vi "gcodeTec.vi"() -> ()   [LabVIEW 2025]
panel:
  out "subarray":dbl[][][](array[numeric])
  out "Array":dbl[][][](array[numeric])
  out "string in":string
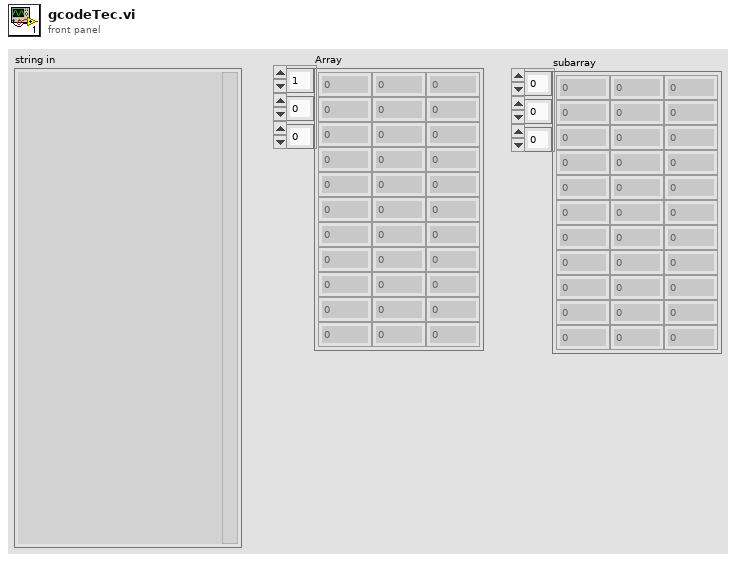
[diagram p1: front panel]
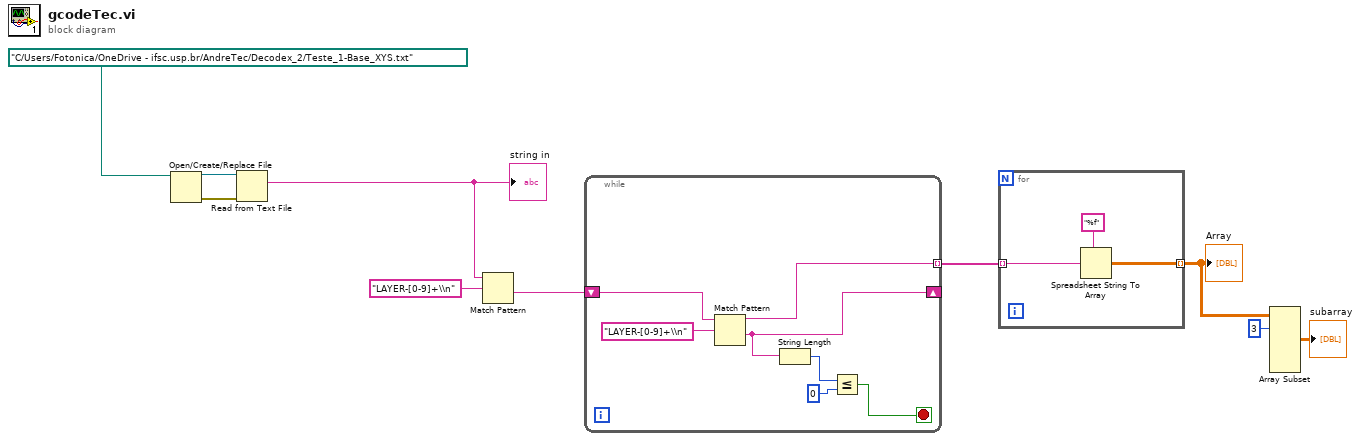
[diagram p0: block diagram]
diagram:
  n1 = Open/Create/Replace File(file path (use dialog)=path "C:/Users/Fotonica/OneDrive - ifsc.usp.br/AndreTec/Decodex_2/Teste_1-Base_XYS.txt") -> (refnum out=w9:refnum<file>, error out=w10:errorcluster)  [unwired: 5 in, 1 out]
  n2 = Read from Text File(file (use dialog)=w9, error in=w10) -> (text=w7:string)  [unwired: 2 in, 3 out]
  "string in" <- w7
  n3 = Match Pattern(string=w7, regular expression="LAYER-[0-9]+\\n") -> (after substring=w5:string)  [unwired: 1 in, 3 out]
  n4 = while {
    shift-right: [w14] -> _
    shift-left: w5 -> [w16]
    tunnel: [w11] -> w4 mode=indexing
    stop <- w12 stop-if-true
    n5 = Match Pattern(string=w16, regular expression="LAYER-[0-9]+\\n") -> (before substring=w11:string, after substring=w14:string)  [unwired: 1 in, 2 out]
    n6 = String Length(string=w14) -> (length=w15:i32)
    n7 = Less Or Equal?(x=w15, y=0) -> (x <= y?=w12:bool)
  }
  n8 = for {
    tunnel: w4 -> [w20] mode=indexing
    tunnel: [w18] -> w3 mode=indexing
    n9 = Spreadsheet String To Array(format string="%f", spreadsheet string=w20) -> (array=w18:dbl[][])  [unwired: 2 in]
  }
  "Array" <- w3
  n10 = Array Subset(array=w3, index (dim 0)=3 ("index")) -> (→"subarray":dbl[][][])  [unwired: 5 in]
